vi "PH_PP_CurrentMeas.PC read RT Client 2.vi"(0 "i ref in":refnum<vi>, 5 "error in (no error)":errorcluster) -> (14 "i ref out":refnum<vi>, 16 "Data PU 4":waveform(dbl)[](array[waveform]), 17 "Data PU 5":waveform(dbl)[](array[waveform]), 18 "Data PU 3":waveform(dbl)[](array[waveform]), 19 "error out":errorcluster)   [LabVIEW 2014, in "PH_PP_CurrentMeas.lvlib"]
doc: "This VI reads out the data of RT client 2."
uses:
  PH_PP_CurrentMeas.lvlib
panel:
  in  "Array":waveform(dbl)[](array[waveform])
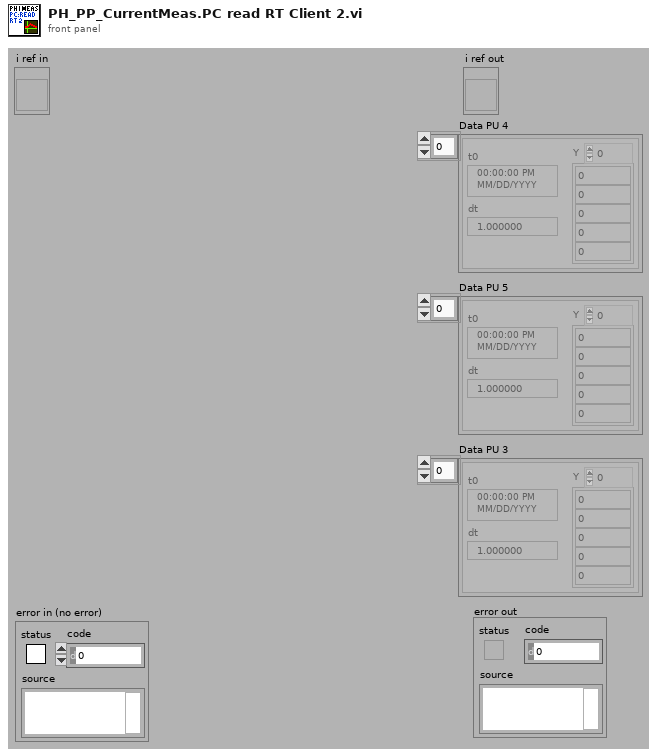
[diagram p1: front panel]
types:
  T1 = typedef "PH_PP_CurrentMeas.lvlib/PH_PP_CurrentMeas.i attribute.ctl" = cluster{"Status":cluster{"GUI Ref Hardware Feedback":refnum<vi>, "Tab Control":refnum<vi>}, "PU 1":cluster{"Instance":string, "Status":T2, "Ref Status ":refnum<vi>, "Data":waveform(dbl)[], "Ref Data":refnum<vi>}, "PU 2":cluster{"Instance":string, "Status":T2, "Ref Status ":refnum<vi>, "Data":waveform(dbl)[], "Ref Data":refnum<vi>}, "PU 3":cluster{"Instance":string, "Status":T2, "Ref Status ":refnum<vi>, "Data":waveform(dbl)[], "Ref Data":refnum<vi>}, "PU 4":cluster{"Instance":string, "Status":T2, "Ref Status ":refnum<vi>, "Data":waveform(dbl)[], "Ref Data":refnum<vi>}, "PU 5":cluster{"Instance":string, "Status":T2, "Ref Status ":refnum<vi>, "Data":waveform(dbl)[], "Ref Data":refnum<vi>}, "FR":cluster{"Instance":string, "Status":T2, "Ref Status ":refnum<vi>, "Data":waveform(dbl)[], "Ref Data":refnum<vi>}, "PA - 19mm 1":cluster{"Instance":string, "Status":T2, "Ref Status ":refnum<vi>}, "PA - 19mm 2":cluster{"Instance":string, "Status":T2, "Ref Status ":refnum<vi>, "no link":bool}, "PA - 45mm":cluster{"Instance":string, "Status":T2, "Ref Status ":refnum<vi>, "no link":bool}, "PA Data":cluster{"Data":waveform(dbl)[], "Ref":refnum<vi>}, "Sequencer":cluster{"Instance":string, "SM State Ref":refnum<vi>}, "Tasks":cluster{"Port":u16, "connection ID":refnum<k5>, "Status":T2, "Ref":refnum<vi>, "Ref Bar":refnum<vi>, "Feedback":cluster{"Received Data Sets":T3[], "Driver Error":errorcluster, "Connection not established":bool, "Error unpacking the data":bool, "No Task defined":bool, "Not triggered yet":bool}, "Data":waveform(dbl)[], "Ref Teststart Task":refnum<vi>}[], "in use":cluster{"MA DP":bool, "FR and PA":bool}, "DAQ Server":string}
  T2 = typedef "PH_StatusHandler.lvlib/PH_StatusHandler.Status.ctl" = i16
  T3 = typedef "PH_PP_CurrentMeas.lvlib/PH_PP_CurrentMeas.CommandCluster.ctl" = cluster{"Command":string, "Data":string, "error out":errorcluster}
  T4 = cluster{"Port":u16, "connection ID":refnum<k5>, "Status":T2, "Ref":refnum<vi>, "Ref Bar":refnum<vi>, "Feedback":cluster{"Received Data Sets":T3[], "Driver Error":errorcluster, "Connection not established":bool, "Error unpacking the data":bool, "No Task defined":bool, "Not triggered yet":bool}, "Data":waveform(dbl)[], "Ref Teststart Task":refnum<vi>}[]
  T5 = cluster{"Port":u16, "connection ID":refnum<k5>, "Status":T2, "Ref":refnum<vi>, "Ref Bar":refnum<vi>, "Feedback":cluster{"Received Data Sets":T3[], "Driver Error":errorcluster, "Connection not established":bool, "Error unpacking the data":bool, "No Task defined":bool, "Not triggered yet":bool}, "Data":waveform(dbl)[], "Ref Teststart Task":refnum<vi>}
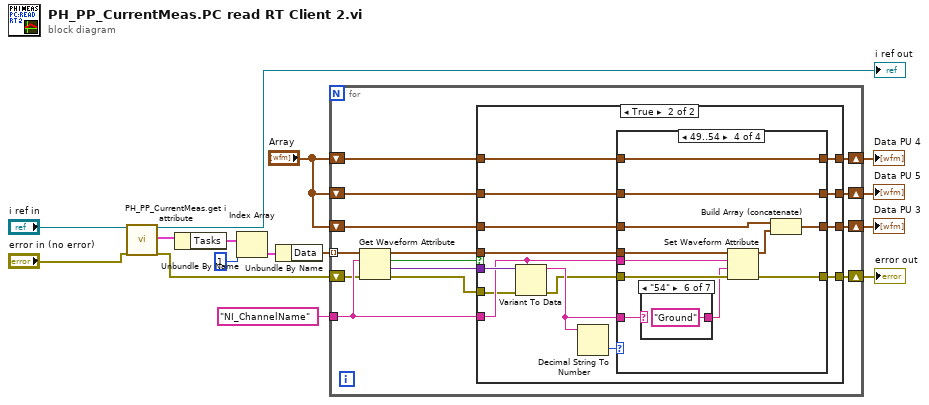
[diagram p0: block diagram]
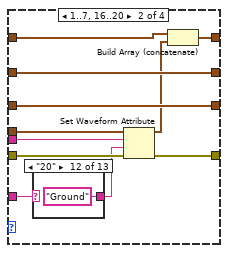
[diagram p4: hidden frame]
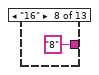
[diagram p12: hidden frame]
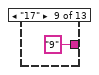
[diagram p13: hidden frame]
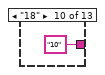
[diagram p14: hidden frame]
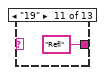
[diagram p15: hidden frame]
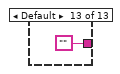
[diagram p16: hidden frame]
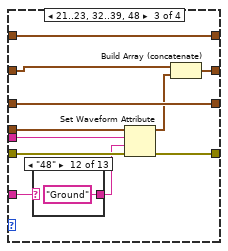
[diagram p17: hidden frame]
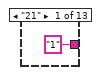
[diagram p18: hidden frame]
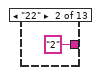
[diagram p19: hidden frame]
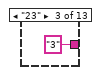
[diagram p20: hidden frame]
diagram:
  n1 = call "PH_PP_CurrentMeas.get i attribute.vi"("i ref in"="i ref in", "error in (no error)"="error in (no error)") -> ("i ref out"=→"i ref out":refnum<vi>, "i attribute"=w15:T1, "error out"=w3:errorcluster)  [unwired: 15 in]
  n2 = Unbundle By Name(w15) -> ("Tasks"=w12:T4)
  n3 = Index Array(array=w12, index=1) -> (element=w2:T5)
  n4 = Unbundle By Name(w2) -> ("Data"=w1:waveform(dbl)[])
  n5 = for {
    tunnel: w1 -> [w20] mode=indexing
    tunnel: "NI_ChannelName" ("name") -> [w21]
    shift-right: [w29] -> w10
    shift-left: w3 -> [w18]
    shift-right: [w28] -> w8
    shift-left: "Array" -> [w27]
    shift-right: [w26] -> w7
    shift-left: "Array" -> [w25]
    shift-right: [w24] -> w6
    shift-left: "Array" -> [w23]
    n6 = Get Waveform Attribute(4:w18, 6:w21, 7:w20) -> (0:w17:errorcluster, 1:w22:variant, 2:w16:bool, 3:w19:waveform(dbl))  [unwired: 1 in]
    n7 = case shown="True" w16 {
      tunnel: w19 -> [_ w47]
      tunnel: w17 -> [w33 w35]
      tunnel: [w33 w46] -> w29
      tunnel: w22 -> [_ w38]
      tunnel: w21 -> [_ w37]
      tunnel: [w32 w44] -> w28
      tunnel: w27 -> [w32 w43]
      tunnel: [w31 w42] -> w26
      tunnel: w25 -> [w31 w41]
      tunnel: [w30 w40] -> w24
      tunnel: w23 -> [w30 w39]
      frame False {
      }
      frame True {
        n8 = Variant To Data(error in=w35, type=w37, Variant=w38) -> (data=w36:string, error out=w34:errorcluster)
        n9 = Decimal String To Number(string=w36) -> (number=w45:i32)  [unwired: 2 in, 1 out]
        n10 = case shown="49..54" w45 {
          tunnel: w47 -> [_ w57 w78 w105]
          tunnel: [w50 w54 w80 w103] -> w46
          tunnel: w37 -> [_ w52 w77 w100]
          tunnel: w34 -> [w50 w55 w81 w102]
          tunnel: [w51 w62 w85 w109] -> w44
          tunnel: w43 -> [w51 w61 w85 w109]
          tunnel: w36 -> [_ w60 w86 w110]
          tunnel: [w49 w59 w84 w108] -> w42
          tunnel: w41 -> [w49 w59 w83 w108]
          tunnel: [w48 w58 w82 w107] -> w40
          tunnel: w39 -> [w48 w58 w82 w106]
          frame Default {
          }
          frame 1..7, 16..20 {
            n11 = case shown="\"20\"" w60 {
              selector: w60 -> [w63 w64 w65 w66 w67 w68 w69 _ _ _ _ _ _]
              tunnel: [w63 w64 w65 w66 w67 w68 w69 "8" "9" "10" "Refl" "Ground" ""] -> w53
              frame "1" {
              }
              frame "2" {
              }
              frame "3" {
              }
              frame "4" {
              }
              frame "5" {
              }
              frame "6" {
              }
              frame "7" {
              }
              frame "16" {
              }
              frame "17" {
              }
              frame "18" {
              }
              frame "19" {
              }
              frame "20" {
              }
              frame Default {
              }
            }
            n12 = Set Waveform Attribute(4:w55, 5:w53, 6:w52, 7:w57) -> (0:w54:errorcluster, 3:w56:waveform(dbl))  [unwired: 1 out]
            n13 = Build Array (concatenate)(w61, w56) -> (w62:waveform(dbl)[])
          }
          frame 21..23, 32..39, 48 {
            n14 = case shown="\"48\"" w86 {
              tunnel: ["1" "2" "3" "4" "5" "6" "7" "8" "9" "10" "Refl" "Ground" ""] -> w76
              frame "21" {
              }
              frame "22" {
              }
              frame "23" {
              }
              frame "32" {
              }
              frame "33" {
              }
              frame "34" {
              }
              frame "35" {
              }
              frame "36" {
              }
              frame "37" {
              }
              frame "38" {
              }
              frame "39" {
              }
              frame "48" {
              }
              frame Default {
              }
            }
            n15 = Set Waveform Attribute(4:w81, 5:w76, 6:w77, 7:w78) -> (0:w80:errorcluster, 3:w79:waveform(dbl))  [unwired: 1 out]
            n16 = Build Array (concatenate)(w83, w79) -> (w84:waveform(dbl)[])
          }
          frame 49..54 {
            n17 = case shown="\"54\"" w110 {
              tunnel: ["7" "8" "9" "10" "Refl" "Ground" ""] -> w101
              frame "49" {
              }
              frame "50" {
              }
              frame "51" {
              }
              frame "52" {
              }
              frame "53" {
              }
              frame "54" {
              }
              frame Default {
              }
            }
            n18 = Set Waveform Attribute(4:w102, 5:w101, 6:w100, 7:w105) -> (0:w103:errorcluster, 3:w104:waveform(dbl))  [unwired: 1 out]
            n19 = Build Array (concatenate)(w106, w104) -> (w107:waveform(dbl)[])
          }
        }
      }
    }
  }
  "error out" <- w10
  "Data PU 4" <- w8
  "Data PU 5" <- w7
  "Data PU 3" <- w6
